vi "Execute Statements.vi"(8 "error in (no error)":errorcluster) -> (0 "error out":errorcluster)   [LabVIEW 2020]
uses:
  G-Embedded-Python-Interpreter-Toolkit/Merge Call Library Errors.vi
  <vilib>/addons/_JKI Toolkits/Caraya/classes/Assert/Assert Equal Value_Variant.vi
  G-Embedded-Python-Interpreter-Toolkit/G-Embedded-Python-Interpreter-Toolkit.lvlib
  <vilib>/addons/_JKI Toolkits/Caraya/classes/Assert/Assert.lvclass
  <vilib>/addons/_JKI Toolkits/Caraya/classes/Test/Test.lvclass
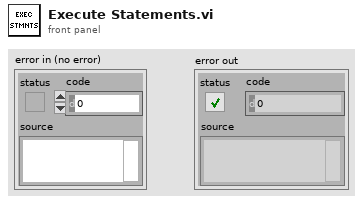
[diagram p1: front panel]
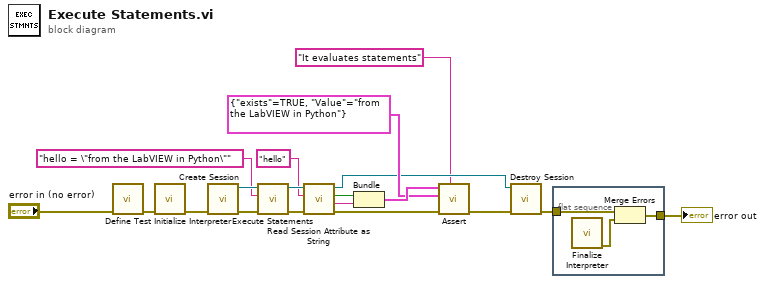
[diagram p0: block diagram]
diagram:
  n1 = call <vilib>:"Define Test.vi"("error in (no error)"="error in (no error)") -> ("error out"=w19:errorcluster)  [unwired: 10 in]
  n2 = call "Initialize Interpreter.vi"("error in (no error)"=w19) -> ("error out"=w16:errorcluster)  [unwired: 9 in, 1 out]
  n3 = call "Create Session.vi"("error in (no error)"=w16) -> ("error out"=w13:errorcluster, "Session Handle"=w15:refnum<data-value>)  [unwired: 9 in]
  n4 = call "Execute Statements.vi"("error in (no error)"=w13, "Statements"="hello = \"from the LabVIEW in Python\"" ("String"), "Session Handle in"=w15) -> ("error out"=w14:errorcluster, "Session Handle out"=w12:refnum<data-value>)  [unwired: 7 in]
  n5 = call "Read Session Attribute as String.vi"("error in (no error)"=w14, "Attribute Name"="hello", "Session Handle in"=w12) -> ("error out"=w8:errorcluster, "Value"=w9:string, "Exists"=w10:bool, "Session Handle out"=w5:refnum<data-value>)  [unwired: 5 in]
  n6 = Bundle("Exists"=w10, "Value"=w9) -> (w7:cluster{"Exists":bool, "Value":string})  [unwired: 1 in]
  n7 = call-poly <vilib>:"Assert.vi"("Label"="It evaluates statements", "error in (no error)"=w8, "Y"=cluster{"exists":bool, "Value":string} {"exists"=TRUE, "Value"="from the LabVIEW in Python"} ("output cluster"), "X"=w7) -> ("error out"=w4:errorcluster)  [unwired: 7 in]
  n8 = call "Destroy Session.vi"("error in (no error)"=w4, "Session Handle"=w5) -> ("error out"=w3:errorcluster)  [unwired: 9 in]
  n9 = flat-sequence {
    tunnel: w3 -> [w22]
    tunnel: [w20] -> w17
    frame #0 {
      n10 = call "Finalize Interpreter.vi"() -> ("error out"=w21:errorcluster)  [unwired: 11 in]
      n11 = Merge Errors(w22, w21) -> (w20:errorcluster)
    }
  }
  "error out" <- w17
